vi "Logger.PGSQL.ReadVariable.vi"(6 "Timeout (ms) [5000]":i32=5000, 8 "error in (no error)":errorcluster, 10 "Address":string, 11 "Logger":refnum<class "Logger.PGSQL.lvclass">) -> (0 "error out":errorcluster, 1 "Data":variant, 3 "Logger out":refnum<class "Logger.PGSQL.lvclass">)   [LabVIEW 2019, in "Logger.PGSQL.lvlib" / "Logger.PGSQL.lvclass"]
doc: "---------------------------------------------------------------\nJKI State Machine Objects™\nhttp://jki.net/state-machine-objects/\nCopyright (C) 2005-2015, JKI <info@jki.net>\nALL RIGHTS RESERVEDJKI State Machine Objects (SMO) 1.0.0.4\nJKI - JKI\nCopyright (c) 2015, JKI"
uses:
  Logger.PGSQL.lvclass
  Typedefs/PrivateEvents--Logger.PGSQL.Read Variable.ctl
  Logger.PGSQL.lvclass/Logger.PGSQL.ctl
  <vilib>/Utility/error.llb/Error Cluster From Error Code.vi
  <vilib>/ErrorRing/Error Ring.xnode
panel:
  # "For instructions on how to use the JKI State Machine Objects, examples and video tutorials, visit:\nhttp://jki.net/state-machine-objects/\n\nJKI State Machine Objects™\nhttp://jki.net/state-machine-objects/\nCopyright (C) 2005-2015, JKI <info@jki.net>\nALL RIGHTS RESERVED"
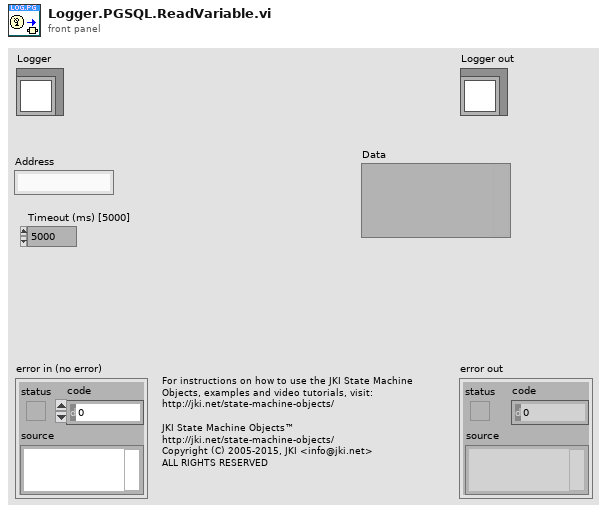
[diagram p1: front panel]
types:
  T1 = typedef "Logger.PGSQL.lvlib/Logger.PGSQL.lvclass/PrivateEvents--Logger.PGSQL.Read Variable.ctl" = cluster{"Address":string}
  T2 = typedef "Logger.PGSQL.lvlib/Logger.PGSQL.lvclass/PublicEvents--Cluster.ctl" = cluster{"Read Variable":refnum<user-event>}
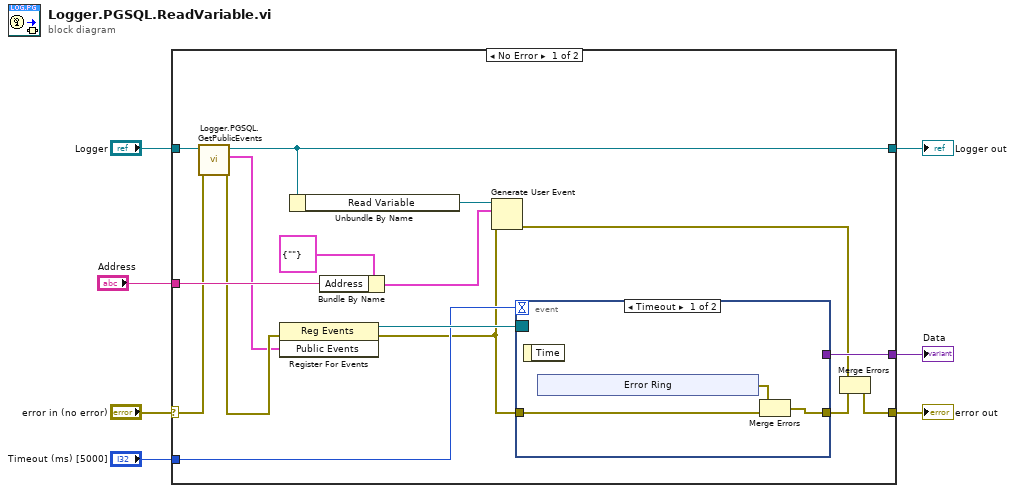
[diagram p0: block diagram]
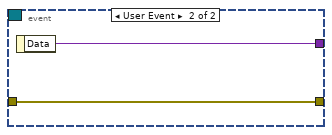
[diagram p2: hidden frame]
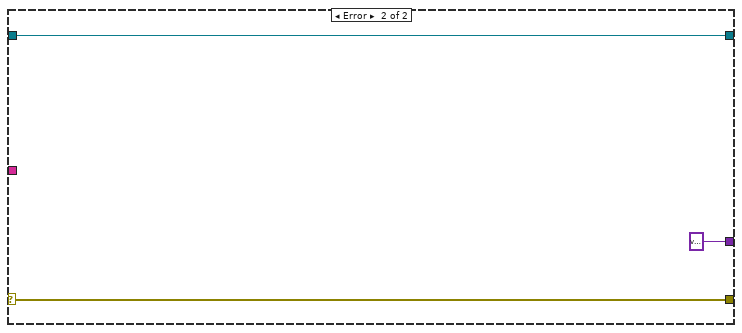
[diagram p3: hidden frame]
diagram:
  n1 = case shown="No Error" "error in (no error)" {
    selector: "error in (no error)" -> [w18 w35]
    tunnel: [w8 w35] -> w6
    tunnel: [w20 w34] -> w7
    tunnel: "Logger" -> [w19 w34]
    tunnel: "Address" -> [w22 _]
    tunnel: "Timeout (ms) [5000]" -> [w16 _]
    tunnel: [w15 variant ("Data")] -> w1
    frame No Error {
      n2 = call "Logger.PGSQL.GetPublicEvents.vi"("error in (no error)"=w18, "Logger"=w19) -> ("error out"=w14:errorcluster, "Public Events"=w13:T2, "Logger out"=w20:refnum<class "Logger.PGSQL.lvclass">)  [unwired: 7 in]
      n3 = register-events(error in=w14, w13) -> (reference out=w17:refnum<event-registration>, error out=w11:errorcluster)  [unwired: 1 in]
      n4 = Unbundle By Name(w20) -> ("Read Variable"=w23:refnum<user-event>)
      n5 = Bundle By Name(cluster=T1 {"Address"=""} ("Read Variable"), "Address"=w22) -> (w12:T1)
      n6 = Generate User Event(user event=w23, event data cluster=w12, error in=w11) -> (error out=w10:errorcluster)  [unwired: 1 in, 1 out]
      n7 = event shown="[0] Timeout" {
        selector: w17 -> [_ _]
        dyn-events: _ -> [_ _]
        timeout: w16 -> [_ _]
        tunnel: [_ w32] -> w15
        tunnel: w11 -> [w25 w31]
        tunnel: [w26 w31] -> w9
        event Timeout {
          n8 = event-data() -> ()  [unwired: 1 in, 1 out]
          n9 = xnode "Error Ring"() -> ("error out"=w24:errorcluster)
          n10 = Merge Errors(w24, w25) -> (w26:errorcluster)
        }
        event User Event {
          n11 = event-data() -> ("Data"=w32:variant)  [unwired: 1 in]
        }
      }
      n12 = Merge Errors(w10, w9) -> (w8:errorcluster)
    }
    frame Error {
    }
  }
  "error out" <- w6
  "Logger out" <- w7
  "Data" <- w1
